vi "Request Notifications.vi"(8 "error in (no error)":errorcluster, 11 "Client - Data In":T1) -> (0 "error out":errorcluster, 3 "Client - Data Out":T1)   [LabVIEW 2024]
doc: "Requests the value change notifications and alarm and event notifications."
uses:
  Controls/Client/Client - Data.ctl
  Shared/Message Queue/Client Message Queues.ctl
  Shared/Message Queue/Message Cluster.ctl
  <vilib>/lvdsc/NI_DSC.lvlib
  Shared/Message Queue.lvlib
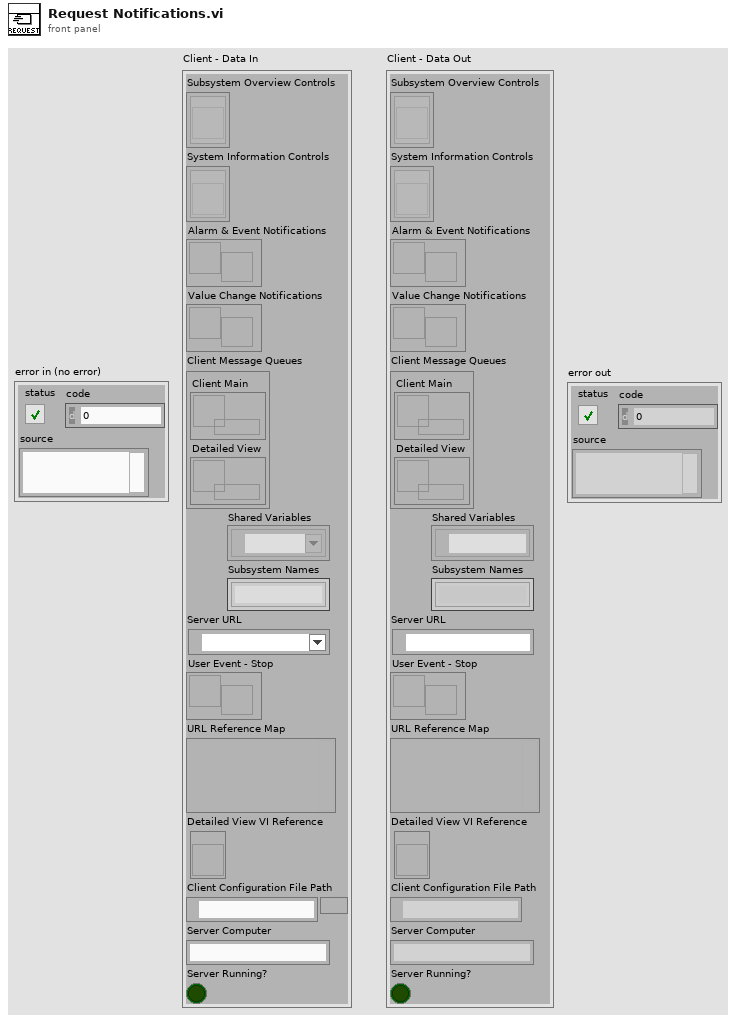
[diagram p1: front panel]
types:
  T1 = typedef "Client - Data.ctl" = cluster{"Subsystem Overview Controls":refnum<vi>[], "System Information Controls":refnum<vi>[], "Alarm & Event Notifications":refnum<user-event>, "Value Change Notifications":refnum<user-event>, "Client Message Queues":T2, "Shared Variables":refnum<k21>[], "Subsystem Names":string[], "Server URL":refnum<k21>, "User Event - Stop":refnum<user-event>, "URL Reference Map":variant, "Detailed View VI Reference":refnum<vi>, "Client Configuration File Path":path, "Server Computer":string, "Server Running?":bool}
  T2 = typedef "Message Queue.lvlib/Client Message Queues.ctl" = cluster{"Client Main":refnum<queue>, "Detailed View":refnum<queue>}
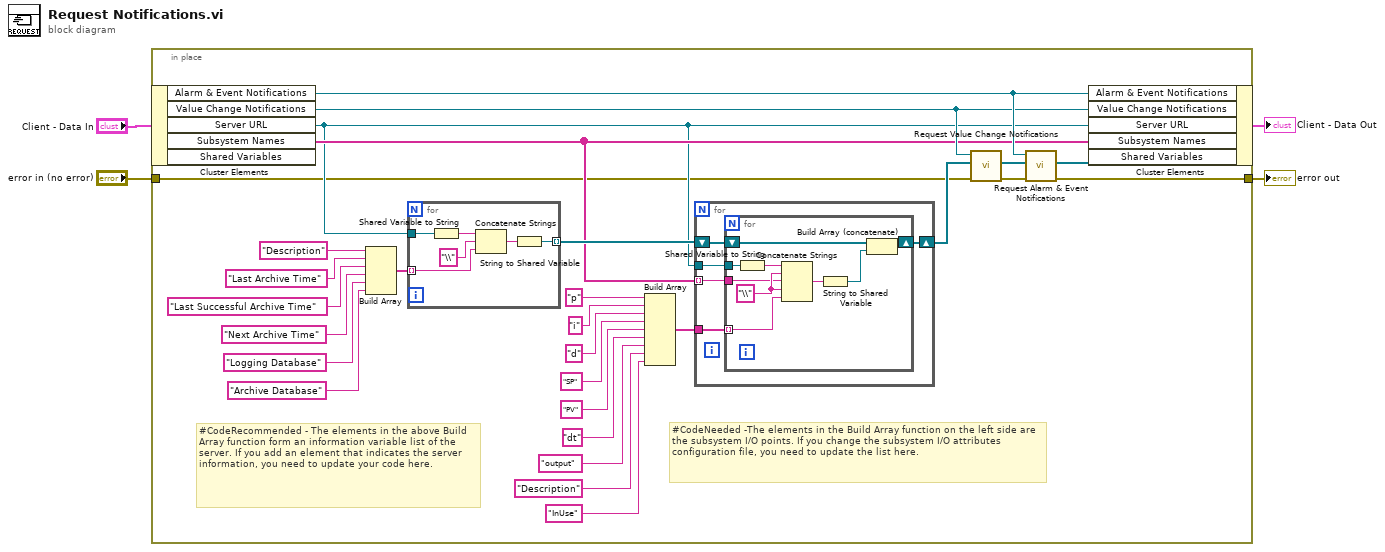
[diagram p0: block diagram]
diagram:
  n1 = in-place {
    in-place-border: [w28] -> w1
    in-place-border: "error in (no error)" -> [w5]
    # "#CodeRecommended - The elements in the above Build Array function form an information variable list of the server. If you add an element that indicates the server information, you need to update your code here."
    # "#CodeNeeded -The elements in the Build Array function on the left side are the subsystem I/O points. If you change the subsystem I/O attributes configuration file, you need to update the list here."
    n2 = in-place-cluster #1("Client - Data In") -> ("Alarm & Event Notifications"=w30:refnum<user-event>, "Value Change Notifications"=w29:refnum<user-event>, "Server URL"=w6:refnum<k21>, "Subsystem Names"=w17:string[])  [unwired: 1 out]
    n3 = Build Array("Description" ("format string"), "Last Archive Time" ("format string"), "Last Successful Archive Time" ("format string"), "Next Archive Time" ("format string"), "Logging Database" ("format string"), "Archive Database" ("format string")) -> (w21:string[])
    n4 = for {
      tunnel: w6 -> [w50]
      tunnel: [w48] -> w20 mode=indexing
      tunnel: w21 -> [w49] mode=indexing
      n5 = Shared Variable to String(1:w50) -> (0:w52:string)
      n6 = Concatenate Strings(w52, "\\" ("string"), w49) -> (w47:string)
      n7 = String to Shared Variable(0:w47) -> (2:w48:refnum<k21>)  [unwired: 1 out]
    }
    n8 = Build Array("p" ("format string"), "i" ("format string"), "d" ("format string"), "SP" ("format string"), "PV" ("format string"), "dt" ("format string"), "output" ("format string"), "Description" ("format string"), "InUse" ("format string")) -> (w7:string[])
    n9 = for {
      shift-right: [w36] -> w19
      shift-left: w20 -> [w37]
      tunnel: w17 -> [w33] mode=indexing
      tunnel: w7 -> [w35]
      tunnel: w6 -> [w34]
      n10 = for {
        shift-right: [w45] -> w36
        shift-left: w37 -> [w46]
        tunnel: w35 -> [w40] mode=indexing
        tunnel: w34 -> [w42]
        tunnel: w33 -> [w39]
        w41 = "\\" ("string")
        n11 = Shared Variable to String(1:w42) -> (0:w43:string)
        n12 = Concatenate Strings(w43, w41, w39, w41, w40) -> (w44:string)
        n13 = String to Shared Variable(0:w44) -> (2:w38:refnum<k21>)  [unwired: 1 out]
        n14 = Build Array (concatenate)(w46, w38) -> (w45:refnum<k21>[])
      }
    }
    n15 = call <vilib>:"Request Value Change Notifications.vi"("error in (no error)"=w5, "shared variables"=w19, "notification refnum"=w29) -> ("error out"=w31:errorcluster, "shared variables out"=w32:refnum<k21>[])  [unwired: 6 in, 1 out]
    n16 = call <vilib>:"Request Alarm & Event Notifications.vi"("error in (no error)"=w31, "shared variables"=w32, "notification refnum"=w30) -> ("error out"=w28:errorcluster, "shared variables out"=w18:refnum<k21>[])  [unwired: 6 in, 1 out]
    n17 = in-place-cluster #1("Alarm & Event Notifications"=w30, "Value Change Notifications"=w29, "Server URL"=w6, "Subsystem Names"=w17, "Shared Variables"=w18) -> (→"Client - Data Out":T1)
  }
  "error out" <- w1
